vi "Acquired Image.vi"(8 "error in (no error)":errorcluster) -> (0 "error out":errorcluster, 1 "Image":dbl[][](array[numeric]), 2 "Slices":i32, 3 "Channels":i32)   [LabVIEW 2018]
uses:
  SesWrapper/SesWrapper.lvlib
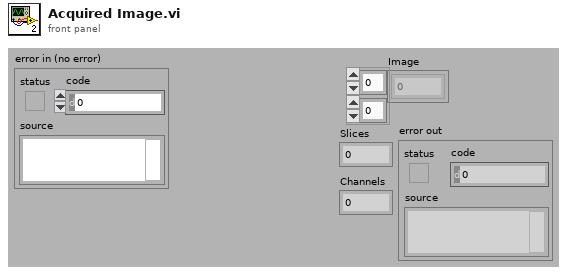
[diagram p1: front panel]
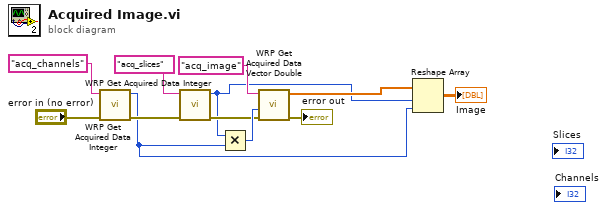
[diagram p0: block diagram]
diagram:
  n1 = call "WRP Get Acquired Data Integer.vi"("error in (no error)"="error in (no error)", "parameter"="acq_channels") -> ("error out"=w8:errorcluster, "data"=w2:i32)  [unwired: 6 in, 2 out]
  n2 = call "WRP Get Acquired Data Integer.vi"("error in (no error)"=w8, "parameter"="acq_slices") -> ("error out"=w7:errorcluster, "data"=w1:i32)  [unwired: 6 in, 2 out]
  n3 = Multiply(x=w1, y=w2) -> (x*y=w9:i32)
  n4 = call "WRP Get Acquired Data Vector Double.vi"("error in (no error)"=w7, "size"=w9, "parameter"="acq_image") -> ("error out"=→"error out":errorcluster, "data"=w5:dbl[])  [unwired: 5 in, 2 out]
  n5 = Reshape Array(w5, w1, w2) -> (→"Image":dbl[][])
